vi "fiji_opener.vi"() -> ()   [LabVIEW 2020]
panel:
  out "error out":errorcluster
  in  "File Path":path=path "C:/Program Files (x86)/fiji-win64/Fiji.app"
  in  "error in (no error)":errorcluster
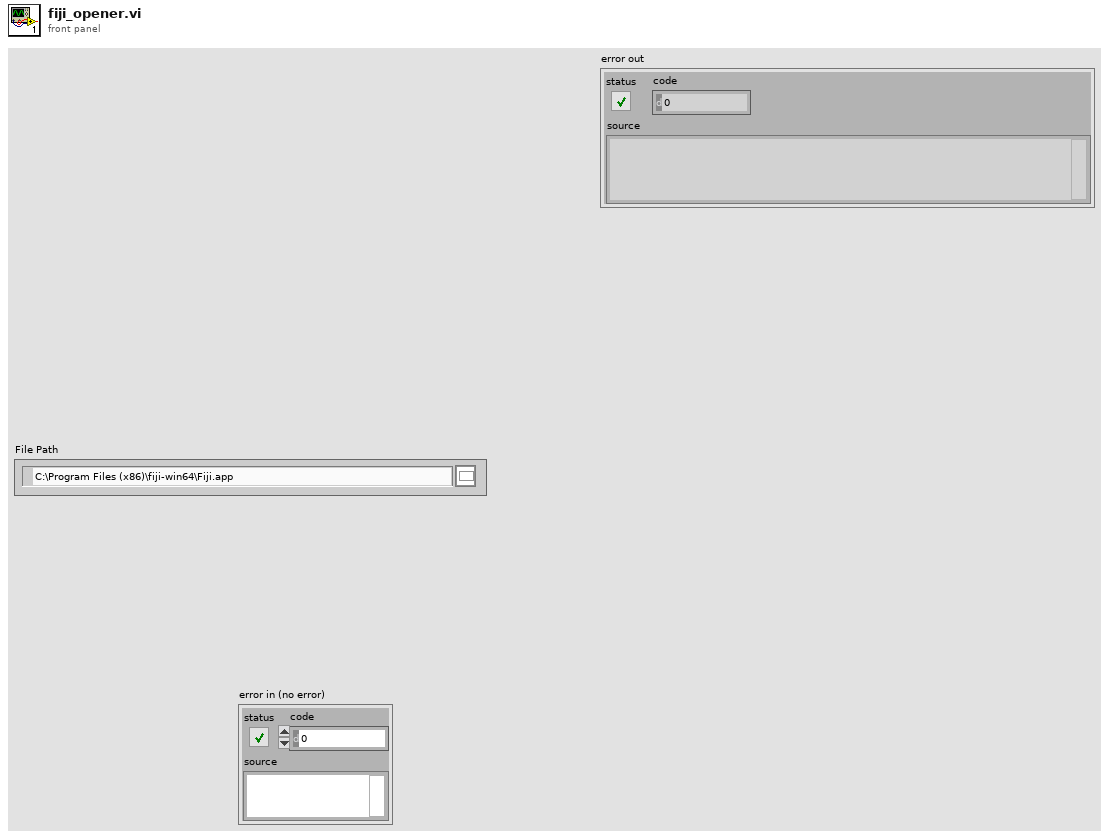
[diagram p1: front panel]
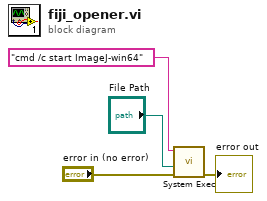
[diagram p0: block diagram]
diagram:
  n1 = call <vilib>:"System Exec.vi"("error in (no error)"="error in (no error)", "working directory"="File Path", "command line"="cmd /c start ImageJ-win64") -> ("error out"=→"error out":errorcluster)  [unwired: 5 in, 3 out]
